vi "produceTimingTick.vi"(8 "error in (no error)":errorcluster, 10 "Channel":refnum<class "Channel.lvclass">, 11 "ScriptEventList in":refnum<class "ScriptEventList.lvclass">) -> (0 "error out":errorcluster, 2 "timingTick":refnum<class "ScriptEventList.lvclass">, 3 "ScriptEventList out":refnum<class "ScriptEventList.lvclass">)   [LabVIEW 2011, in "Tools.lvlib" / "Scripting.lvlib" / "ScriptEventList.lvclass"]
uses:
  ScriptEventList.lvclass
  DatabaseHelpers/Database Objects/Channel/Channel.lvclass
  ScriptEventList.lvclass/ScriptEventList.ctl
  ScriptEvent.lvclass
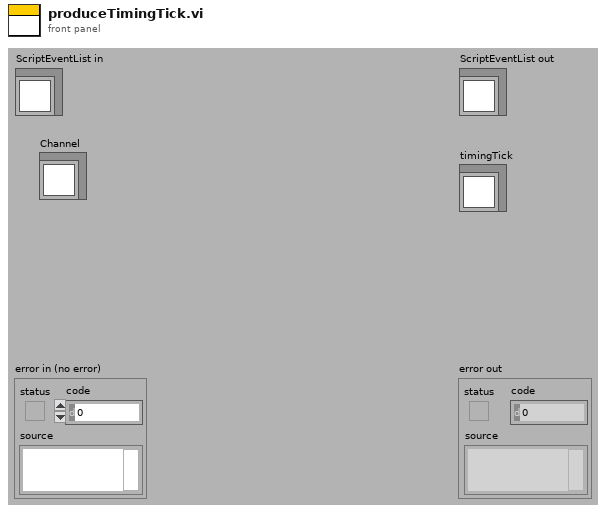
[diagram p1: front panel]
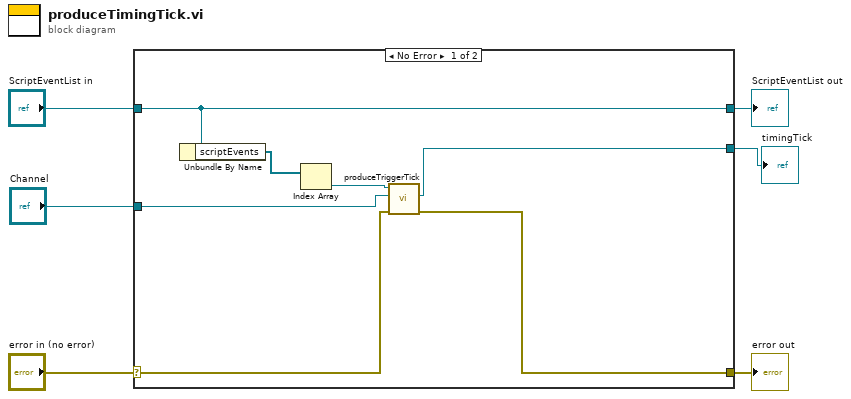
[diagram p0: block diagram]
diagram:
  n1 = case shown="No Error" "error in (no error)" {
    selector: "error in (no error)" -> [w7 w15]
    tunnel: [w10 w15] -> w5
    tunnel: [w13 w14] -> w3
    tunnel: "ScriptEventList in" -> [w13 w14]
    tunnel: "Channel" -> [w11 _]
    tunnel: [w8 _] -> w1
    frame No Error {
      n2 = Unbundle By Name(w13) -> ("scriptEvents"=w12:refnum<class "ScriptEvent.lvclass">[])
      n3 = Index Array(array=w12) -> (element=w9:refnum<class "ScriptEvent.lvclass">)  [unwired: 1 in]
      n4 = call-dynamic "produceTriggerTick.vi"("error in (no error)"=w7, "Channel"=w11, "ScriptEvent in"=w9) -> ("error out"=w10:errorcluster, "timingTick"=w8:refnum<class "ScriptEventList.lvclass">)  [unwired: 6 in, 1 out]
    }
    frame Error {
    }
  }
  "error out" <- w5
  "ScriptEventList out" <- w3
  "timingTick" <- w1
